vi "Open Encoder.vi"   [LabVIEW 2020]
uses:
  <vilib>/Rock Robotics/SystemInterfaces/AI/FPGA_AIChannel.ctl
  <vilib>/Rock Robotics/SystemInterfaces/DIO/FPGA_DIOChannel.ctl
  <vilib>/Rock Robotics/WPI/Counter/WPI_CounterDigitalInputToDigitalSource.vi
  <vilib>/Rock Robotics/WPI/Counter/WPI_CounterOpen UpDown Mode.vi
types:
  T1 = typedef "FPGA_AIChannel.ctl" = enum8{"AI 0", "AI 1", "AI 2", "AI 3", "AI MXP 0", "AI MXP 1", "AI MXP 2", "AI MXP 3", "Invalid"}
  T2 = typedef "FPGA_DIOChannel.ctl" = enum8{"DIO 0", "DIO 1", "DIO 2", "DIO 3", "DIO 4", "DIO 5", "DIO 6", "DIO 7", "DIO 8", "DIO 9", "DIO MXP 0", "DIO MXP 1", "DIO MXP 2", "DIO MXP 3", "DIO MXP 4", "DIO MXP 5", "DIO MXP 6", "DIO MXP 7", "DIO MXP 8", "DIO MXP 9", "DIO MXP 10", "DIO MXP 11", "DIO MXP 12", "DIO MXP 13", "DIO MXP 14", "DIO MXP 15", "SPI Port CS1", "SPI Port CS2", "SPI Port CS3", "SPI Port MISO", "SPI Port MOSI", "Invalid"}
  T3 = typedef "WPI_DigitalInputDevRef.ctl" = cluster{"DevStatus":errorcluster, "DIO Channel":T2}
  T4 = typedef "FPGA_CounterEncoderSourceConvertionLVSourceType.ctl" = cluster{"DevStatus":errorcluster, "AnalogTriggerMode?":bool, "DigitalMode":cluster{"DIO Channel":T5}, "AnalogTriggerMode":cluster{"AnalogTriggerIndex":T6, "OutputType":T7}}
  T5 = typedef "FPGA_DIODigitalSourceChannel.ctl" = enum8{"DIO 0", "DIO 1", "DIO 2", "DIO 3", "DIO 4", "DIO 5", "DIO 6", "DIO 7", "DIO 8", "DIO 9", "DIO MXP 0", "DIO MXP 1", "DIO MXP 2", "DIO MXP 3", "DIO MXP 4", "DIO MXP 5", "DIO MXP 6", "DIO MXP 7", "DIO MXP 8", "DIO MXP 9", "DIO MXP 10", "DIO MXP 11", "DIO MXP 12", "DIO MXP 13", "DIO MXP 14", "DIO MXP 15", "SPI Port CS1", "SPI Port CS2", "SPI Port CS3", "SPI Port MISO", "SPI Port MOSI", "Disabled"}
  T6 = typedef "FPGA_AnalogTriggerIndex.ctl" = enum8{"Trig 0", "Trig 1", "Trig 2", "Trig 3", "Trig 4", "Trig 5", "Trig 6", "Trig 7", "Invalid"}
  T7 = typedef "FPGA_AnalogTriggerOutType.ctl" = enum16{"InWindow", "TriggerState", "Rising", "Falling"}
  T8 = typedef "WPI_CounterDevRef.ctl" = cluster{"DevStatus":errorcluster, "CntIndex":T9}
  T9 = typedef "FPGA_CounterCtrSystemIndex.ctl" = enum8{"Ctr 0", "Ctr 1", "Ctr 2", "Ctr 3", "Ctr 4", "Ctr 5", "Ctr 6", "Ctr 7", "Invalid"}
  T10 = typedef "WPI_AnalogChannelDevRef.ctl" = cluster{"DevStatus":errorcluster, "Analog Channel":T1}
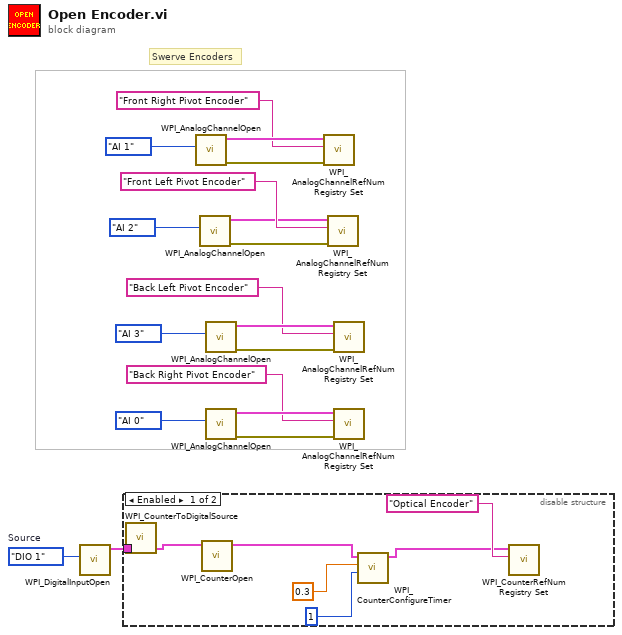
[diagram p0: block diagram]
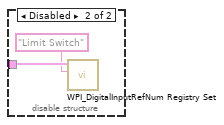
[diagram p2: hidden frame]
diagram:
  w14 = FPGA_DIOChannel."DIO 1"  # Source
  # "Swerve Encoders"
  n1 = call <vilib>:"WPI_DigitalInputOpen.vi"("DIO Channel"=w14) -> ("DigitalInputDevRef"=w13:T3)  [unwired: 1 in, 9 out]
  n2 = disable-structure shown="Enabled" {
    disable-tunnel: w13 -> [w24 w27]
    frame Enabled {
      n3 = call-poly <vilib>:"WPI_CounterToDigitalSource.vi"("DigitalInputDevRef"=w24) -> ("Digital Source"=w25:T4)  [unwired: 6 out]
      n4 = call-poly <vilib>:"WPI_CounterOpen.vi"("Up Source"=w25) -> ("CounterDevRef"=w21:T8)  [unwired: 6 in, 4 out]
      n5 = call <vilib>:"WPI_CounterConfigureTimer.vi"("Number Samples to Average"=1, "MaxPeriod (sec)"=0.3, "CounterDevRef in"=w21) -> ("CounterDevRef out"=w22:T8)  [unwired: 7 in, 1 out]
      n6 = call <vilib>:"WPI_CounterRefNum Registry Set.vi"("refnum name"="Optical Encoder", "CounterDevRef"=w22) -> ()  [unwired: 8 in, 2 out]
    }
    frame Disabled {
      n7 = call <vilib>:"WPI_DigitalInputRefNum Registry Set.vi"("refnum name"="Limit Switch", "DigitalInputDevRef"=w27) -> ()  [unwired: 8 in, 2 out]
    }
  }
  n8 = call <vilib>:"WPI_AnalogChannelOpen.vi"("Analog Channel"=FPGA_AIChannel."AI 1") -> ("error out"=w16:errorcluster, "AIDeviceRef"=w18:T10)  [unwired: 9 in]
  n9 = call <vilib>:"WPI_AnalogChannelOpen.vi"("Analog Channel"=FPGA_AIChannel."AI 2") -> ("error out"=w11:errorcluster, "AIDeviceRef"=w9:T10)  [unwired: 9 in]
  n10 = call <vilib>:"WPI_AnalogChannelOpen.vi"("Analog Channel"=FPGA_AIChannel."AI 3") -> ("error out"=w6:errorcluster, "AIDeviceRef"=w8:T10)  [unwired: 9 in]
  n11 = call <vilib>:"WPI_AnalogChannelOpen.vi"("Analog Channel"=FPGA_AIChannel."AI 0") -> ("error out"=w2:errorcluster, "AIDeviceRef"=w4:T10)  [unwired: 9 in]
  n12 = call <vilib>:"WPI_AnalogChannelRefNum Registry Set.vi"("error in (no error)"=w16, "refnum name"="Front Right Pivot Encoder", "AIDeviceRef"=w18) -> ()  [unwired: 7 in, 2 out]
  n13 = call <vilib>:"WPI_AnalogChannelRefNum Registry Set.vi"("error in (no error)"=w11, "refnum name"="Front Left Pivot Encoder", "AIDeviceRef"=w9) -> ()  [unwired: 7 in, 2 out]
  n14 = call <vilib>:"WPI_AnalogChannelRefNum Registry Set.vi"("error in (no error)"=w6, "refnum name"="Back Left Pivot Encoder", "AIDeviceRef"=w8) -> ()  [unwired: 7 in, 2 out]
  n15 = call <vilib>:"WPI_AnalogChannelRefNum Registry Set.vi"("error in (no error)"=w2, "refnum name"="Back Right Pivot Encoder", "AIDeviceRef"=w4) -> ()  [unwired: 7 in, 2 out]
